vi "GE_BinFile.vi"(0 "refnum":refnum<file>) -> (4 "refnum out":refnum<file>, 6 "# lines per scan":i32, 8 "sample rate":u16, 10 "# rf points per line":u16, 13 "Scan Settings":T2 {"prf (kHz)" format="%.2f"; "Gain (db)" items=["26.0", "40.0", "54.0"]; "LP Filt (MHz)" items=["20", "50", "100", "200"]; "HP Filt(KHz)" items=["1", "1000", "3000", "10000"]; "Damping (In Ohm)" items=["7", "10", "16", "20", "26", "30", "40", "50"]; "Energy (microJ)" items=["1", "2", "4", "8", "16", "32"]}, 15 "Header In":T1={"header info"={"Header"="", "Head length"=0}, "A/D info"={"# rf points per line"=0, "# lines per scan"=0, "sample rate MHz"=0, "# A/D bits"=0, "# bytes per A/D"=0, "TGC Flag"=0, "A/D Type"=""}, "Tranducer Info"={"bandwidth"=0.0, "center freq"=0.0, "start freq"=0.0, "ID"=0}, "Scan Info"={"delay"=0.0, "pivot distance"=0.0, "sector scan angle"=0.0, "operator"="", "Scan Mode"="", "location"=""}, "Time/Date Info"={"date"="", "time"=""}, "RF Info"={"RF file name"="", "RF file att"="", "RF cal file name"="", "RF cal file att"=""}, "Patient Info"={"ID"="", "extended ID"="", "age"=0, "sex"="", "previously\nscanned"="", "PSA"=0.0, "LOS"=1, "Ethnicty 2"=3, "Race"=3}, "Tissue Type"={"organ"=0, "disease type"=0, "disease location"=0, "IQ_pts"=0, "RcvBuffer"=0, "RcvFrame"=0, "IQBuff"=0, "IQFrame"=0, "IQPage"=0}, "Votage scaling"={"Digitizer (dB)"=0.0, "Gain (dB)"=0.0, "Atten (dB)"=0.0}, "Comment"="", "Misc Info"={"avg num"=0, "c speed"=0, "Div By or SF zones"=0, "XMIT CHS"=0, "RCV CHS"=0, "Xmit angle"=0.0}, "Therapy Parameters"={"Theraputic Freq (MHz)"=0.1, "Time on (s)"=1.0, "Therapy amplitude (mV)"=50.0, "Lines Before"=20, "Lines After"=80}, "Scan Settings"={"Energy (uJ or V)"=0, "Damp (Ohm) or Fc"=0, "HP Filt (KHz)"=0, "LP Filt (MHz)"=0, "Gain (db)"=0, "prf (kHz)"=0.0, "Distance between\nscan lines (um)"=0, "Distance between\nscan planes (um)"=0, "Scan line gap (um)"=0.0, "Scan plane gap (um)"=0.0}, "Compression Parameters"={"F1 (MHz)"=0.0, "F2 (MHz)"=0.0, "% taper"=0.0, "duration"=0.0}, "Patient Info Xtra"={"First Name"="", "Last Name"="", "Notes"=""}, "ROI Box"=[]} {"Compression Parameters"."% taper" min=50 max=1000 format="%.2f"; "Compression Parameters"."F2 (MHz)" format="%.3f"; "Compression Parameters"."F1 (MHz)" format="%.3f"; "Scan Settings"."prf (kHz)" format="%.2f"; "Therapy Parameters"."Therapy amplitude (mV)" min=50 max=1000 format="%.2f"; "Therapy Parameters"."Time on (s)" format="%.3f"; "Therapy Parameters"."Theraputic Freq (MHz)" format="%.3f"; "Patient Info"."Race" items=["Am Ind or Alaska", "Asian", "Hawaiian, Pac Isl", "Black or Afr Amer", "White", "more than one race", "unknown"]; "Patient Info"."Ethnicty 2" items=["Hispanic", "Non-Hispanic", "unknown"]; "Patient Info"."LOS" items=["1", "2", "3", "4", "5"]; "Patient Info"."PSA" format="%.1f"; "Scan Info"."delay" format="%.2f"; "Scan Info"."pivot distance" format="%.2f"; "Scan Info"."sector scan angle" format="%.2f"; "Tranducer Info"."bandwidth" format="%.2f"; "Tranducer Info"."center freq" format="%.2f"; "Tranducer Info"."start freq" format="%.2f"})   [LabVIEW 2022 SP3]
uses:
  Header.ctl
panel:
  out "A/D info":T3={"# rf points per line"=0, "# lines per scan"=0, "sample rate MHz"=0, "# A/D bits"=8, "# bytes per A/D"=1, "TGC Flag"=0, "A/D Type"=""}
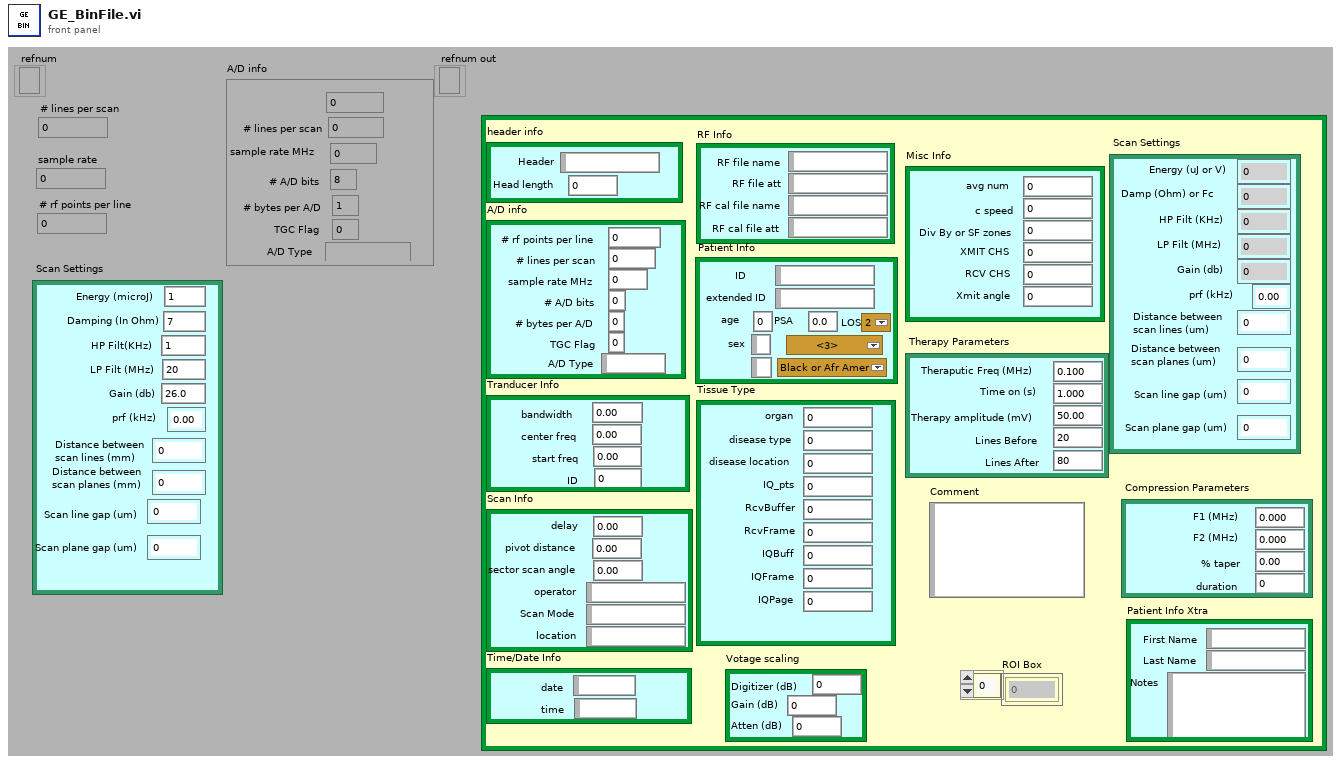
[diagram p1: front panel]
types:
  T1 = typedef "Header.ctl" = cluster{"header info":cluster{"Header":string, "Head length":i16}, "A/D info":cluster{"# rf points per line":u16, "# lines per scan":u16, "sample rate MHz":u16, "# A/D bits":i16, "# bytes per A/D":u16, "TGC Flag":u16, "A/D Type":string}, "Tranducer Info":cluster{"bandwidth":sgl, "center freq":sgl, "start freq":sgl, "ID":i32}, "Scan Info":cluster{"delay":sgl, "pivot distance":sgl, "sector scan angle":sgl, "operator":string, "Scan Mode":string, "location":string}, "Time/Date Info":cluster{"date":string, "time":string}, "RF Info":cluster{"RF file name":string, "RF file att":string, "RF cal file name":string, "RF cal file att":string}, "Patient Info":cluster{"ID":string, "extended ID":string, "age":u16, "sex":string, "previously\nscanned":string, "PSA":sgl, "LOS":u8, "Ethnicty 2":u8, "Race":u8}, "Tissue Type":cluster{"organ":i16, "disease type":i16, "disease location":i16, "IQ_pts":u16, "RcvBuffer":u8, "RcvFrame":u16, "IQBuff":u8, "IQFrame":u16, "IQPage":u8}, "Votage scaling":cluster{"Digitizer (dB)":sgl, "Gain (dB)":sgl, "Atten (dB)":sgl}, "Comment":string, "Misc Info":cluster{"avg num":u16, "c speed":i16, "Div By or SF zones":i16, "XMIT CHS":u8, "RCV CHS":u8, "Xmit angle":sgl}, "Therapy Parameters":cluster{"Theraputic Freq (MHz)":sgl, "Time on (s)":sgl, "Therapy amplitude (mV)":sgl, "Lines Before":u16, "Lines After":u16}, "Scan Settings":cluster{"Energy (uJ or V)":u8, "Damp (Ohm) or Fc":u8, "HP Filt (KHz)":u8, "LP Filt (MHz)":u8, "Gain (db)":u8, "prf (kHz)":sgl, "Distance between\nscan lines (um)":u16, "Distance between\nscan planes (um)":u16, "Scan line gap (um)":sgl, "Scan plane gap (um)":sgl}, "Compression Parameters":cluster{"F1 (MHz)":sgl, "F2 (MHz)":sgl, "% taper":sgl, "duration":sgl}, "Patient Info Xtra":cluster{"First Name":string, "Last Name":string, "Notes":string}, "ROI Box":u16[]}
  T2 = cluster{"Energy (microJ)":u8, "Damping (In Ohm)":u8, "HP Filt(KHz) ":u8, "LP Filt (MHz)":u8, "Gain (db)":u8, "prf (kHz)":sgl, "Distance between\nscan lines (mm)":u16, "Distance between\nscan planes (mm)":u16, "Scan line gap (um)":sgl, "Scan plane gap (um)":sgl}
  T3 = cluster{"# rf points per line":u16, "# lines per scan":u16, "sample rate MHz":u16, "# A/D bits":i16, "# bytes per A/D":u16, "TGC Flag":u16, "A/D Type":string}
  T4 = cluster{"delay":sgl, "pivot distance":sgl, "sector scan angle":sgl, "operator":string, "Scan Mode":string, "location":string}
  T5 = enum16{"big-endian, network order", "native, host order", "little-endian"}
  T6 = cluster{"Energy (microJ)":u8, "Damping (In Ohm)":u8, "HP Filt(KHz)":u8, "LP Filt (MHz)":u8, "Gain (db)":u8, "prf (kHz)":sgl, "Distance between\nscan lines (mm)":u16, "Distance between\nscan planes (mm)":u16, "Distance between\nscan lines (mm) 2":sgl, "Distance between\nscan planes (mm) 2":sgl}
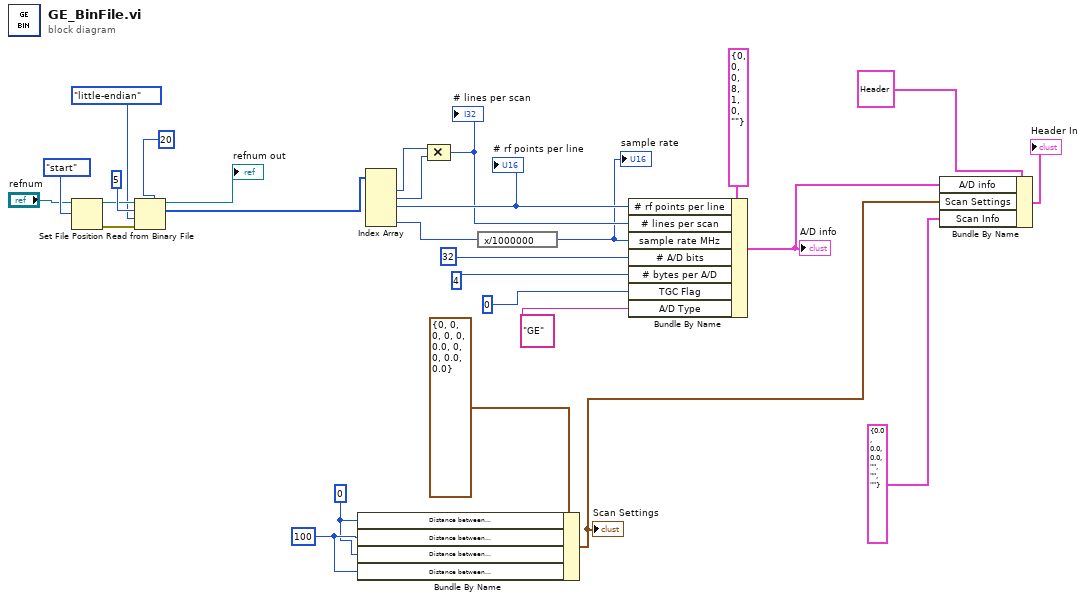
[diagram p0: block diagram]
diagram:
  w2 = u16 100 ("Distance between\nscan planes (mm)")
  w1 = u16 0 ("Distance between\nscan planes (mm)")
  n1 = Set File Position(refnum="refnum", from (0:start)=enum16{"start", "end", "current"}."start" ("pos mode (0:2)")) -> (refnum out=w22:refnum<file>, error out=w21:errorcluster)  [unwired: 1 in, 1 out]
  n2 = Read from Binary File(5:20, 8:w21, 9:T5."little-endian" ("byte order (0:big-endian, network order)"), 10:5, 11:w22) -> (2:w17:i32[], 3:→"refnum out":refnum<file>)  [unwired: 3 out]
  n3 = Bundle By Name(cluster=T6 {"Energy (microJ)"=0, "Damping (In Ohm)"=0, "HP Filt(KHz)"=0, "LP Filt (MHz)"=0, "Gain (db)"=0, "prf (kHz)"=0.0, "Distance between\nscan lines (mm)"=0, "Distance between\nscan planes (mm)"=0, "Distance between\nscan lines (mm) 2"=0.0, "Distance between\nscan planes (mm) 2"=0.0} ("Scan Settings"), "Distance between\nscan planes (mm)"=w1, "Distance between\nscan lines (mm)"=w2, "Distance between\nscan lines (mm) 2"=w1, "Distance between\nscan planes (mm) 2"=w2) -> (w6:T6)
  "Scan Settings" <- w6
  n4 = Index Array(array=w17) -> (element #1=w14:i32, element #2=w13:i32, element #3=w15:i32, element #5=w11:i32)  [unwired: 5 in, 1 out]
  "# rf points per line" <- w15
  n5 = Compound Arithmetic op=MULTIPLY(w14, w13) -> (w12:i32)
  "# lines per scan" <- w12
  n6 = expression code="x/1000000"(w11) -> (w4:i32)
  "sample rate" <- w4
  n7 = Bundle By Name(cluster=T3 {"# rf points per line"=0, "# lines per scan"=0, "sample rate MHz"=0, "# A/D bits"=8, "# bytes per A/D"=1, "TGC Flag"=0, "A/D Type"=""} ("A/D info"), "# rf points per line"=w15, "# lines per scan"=w12, "sample rate MHz"=w4, "# A/D bits"=32, "# bytes per A/D"=4, "TGC Flag"=0, "A/D Type"="GE") -> (w9:T3)
  "A/D info" <- w9
  n8 = Bundle By Name(cluster=T1 {"header info"={"Header"="HEADER_v5.0 ", "Head length"=1024}, "A/D info"={"# rf points per line"=3000, "# lines per scan"=254, "sample rate MHz"=125, "# A/D bits"=14, "# bytes per A/D"=2, "TGC Flag"=0, "A/D Type"="Alaz"}, "Tranducer Info"={"bandwidth"=0.0, "center freq"=0.0, "start freq"=0.0, "ID"=0}, "Scan Info"={"delay"=0.0, "pivot distance"=0.0, "sector scan angle"=0.0, "operator"="    ", "Scan Mode"="A scan ", "location"="RRI      "}, "Time/Date Info"={"date"="0  ", "time"="12:14 PM"}, "RF Info"={"RF file name"="", "RF file att"=".", "RF cal file name"="             ", "RF cal file att"="   "}, "Patient Info"={"ID"="temp  ", "extended ID"="          ", "age"=0, "sex"=" ", "previously\nscanned"=" ", "PSA"=30.0, "LOS"=255, "Ethnicty 2"=0, "Race"=3}, "Tissue Type"={"organ"=2, "disease type"=3, "disease location"=1, "IQ_pts"=0, "RcvBuffer"=0, "RcvFrame"=0, "IQBuff"=0, "IQFrame"=0, "IQPage"=0}, "Votage scaling"={"Digitizer (dB)"=0.0, "Gain (dB)"=0.0, "Atten (dB)"=0.0}, "Comment"="                                                                ", "Misc Info"={"avg num"=1, "c speed"=1485, "Div By or SF zones"=41, "XMIT CHS"=0, "RCV CHS"=0, "Xmit angle"=0.0}, "Therapy Parameters"={"Theraputic Freq (MHz)"=0.0, "Time on (s)"=0.0, "Therapy amplitude (mV)"=0.0, "Lines Before"=0, "Lines After"=0}, "Scan Settings"={"Energy (uJ or V)"=0, "Damp (Ohm) or Fc"=0, "HP Filt (KHz)"=0, "LP Filt (MHz)"=0, "Gain (db)"=0, "prf (kHz)"=0.0, "Distance between\nscan lines (um)"=0, "Distance between\nscan planes (um)"=0, "Scan line gap (um)"=0.0, "Scan plane gap (um)"=0.0}, "Compression Parameters"={"F1 (MHz)"=0.0, "F2 (MHz)"=0.0, "% taper"=0.0, "duration"=0.0}, "Patient Info Xtra"={"First Name"="        ", "Last Name"="                ", "Notes"="                                                                                                                                                                                                   "}, "ROI Box"=[8224, 8224, 8224, 8224]} ("Header In"), "A/D info"=w9, "Scan Settings"=w6, "Scan Info"=T4 {"delay"=0.0, "pivot distance"=0.0, "sector scan angle"=0.0, "operator"="", "Scan Mode"="", "location"=""}) -> (→"Header In":T1)
